vi "Get Data Name.vi"(8 "error in":errorcluster, 11 "Data":refnum<class "variant.lvclass">) -> (0 "error out":errorcluster, 2 "Data Name":string, 3 "Data dup":refnum<class "variant.lvclass">)   [LabVIEW 2020, in "variant.lvlib" / "variant.lvclass"]
doc: "Returns the name of the data wired on input."
uses:
  variant.lvclass
  variant.lvclass/variant.ctl
  Type Descriptor/TD.lvclass
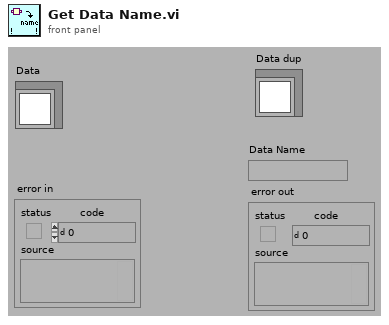
[diagram p1: front panel]
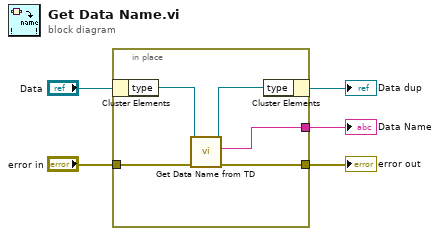
[diagram p0: block diagram]
diagram:
  n1 = in-place {
    in-place-border: [w10] -> w5
    in-place-border: "error in" -> [w9]
    in-place-border: [w8] -> w3
    n2 = in-place-cluster #1("Data") -> ("type"=w7:refnum<class "TD.lvclass">)
    n3 = call "Get Data Name from TD.vi"("error in (no error)"=w9, "TypeDescriptor"=w7) -> ("error"=w10:errorcluster, "name"=w8:string, "TypeDescriptor out"=w6:refnum<class "TD.lvclass">)  [unwired: 7 in]
    n4 = in-place-cluster #1("type"=w6) -> (→"Data dup":refnum<class "variant.lvclass">)
  }
  "error out" <- w5
  "Data Name" <- w3
